vi "CSV to Graph.vi"() -> ()   [LabVIEW 2017]
uses:
  <vilib>/Utility/file.llb/Read Delimited Spreadsheet (DBL).vi
panel:
  out "Waveform Graph":dbl[][](graph)
  in  "File Path Control":path
  out "Error Out":errorcluster
  in  "Error In":errorcluster
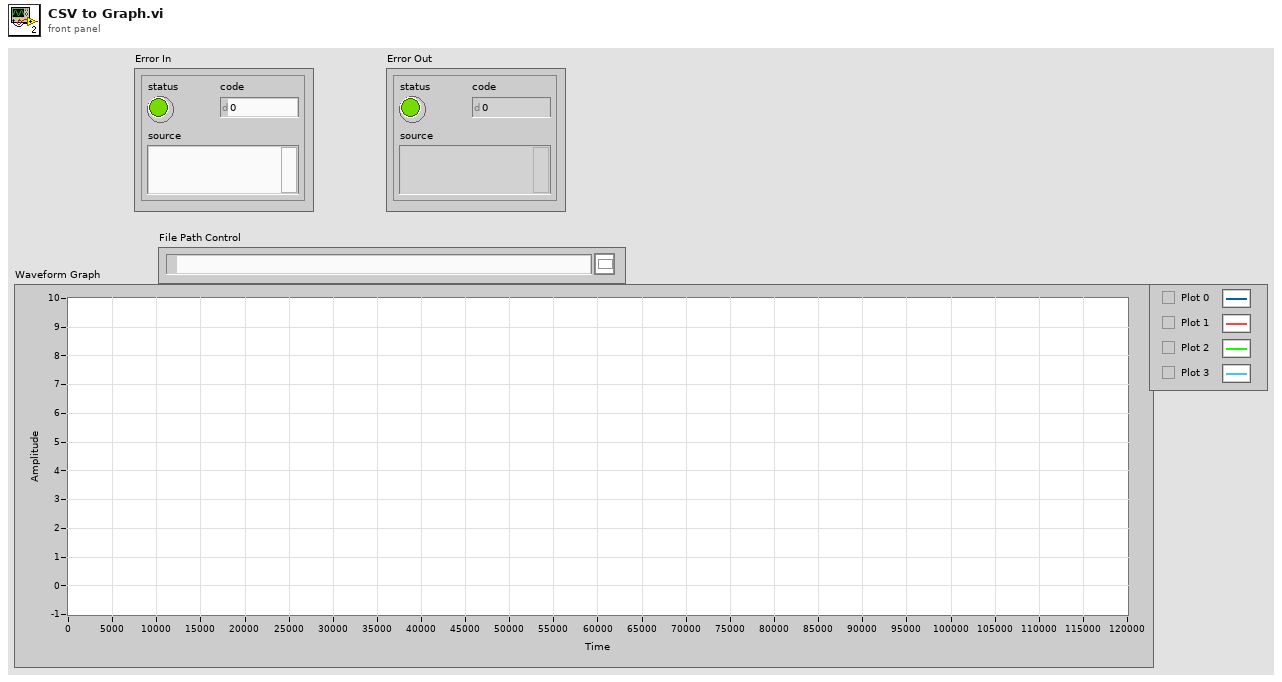
[diagram p1: front panel]
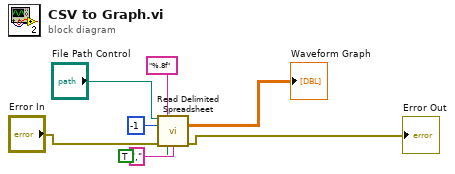
[diagram p0: block diagram]
diagram:
  n1 = call-poly <vilib>:"Read Delimited Spreadsheet.vi"("file path (dialog if empty)"="File Path Control", "format (%.3f)"="%.8f", "number of rows (all:-1)"=-1, "error in (no error)"="Error In", "transpose? (F)"=TRUE, "delimiter (\\t)"="," ("delimiter (\\t)")) -> ("all rows"=→"Waveform Graph":dbl[][], "error out"=→"Error Out":errorcluster)  [unwired: 4 in, 4 out]
